vi "Sub_Initialize_LEMP.vi"(1 "Stiff":T2, 2 "Mass":T2) -> (0 "LEMP":T1)   [LabVIEW 2019]
uses:
  <vilib>/Analysis/Matrix/Datatypes/RealMatrix.ctl
  <vilib>/Analysis/Matrix/Numeric/Conversions/Matrix To Array - RM.vi
  <vilib>/Analysis/Matrix/Numeric/Conversions/Array To Matrix - RA2.vi
  <vilib>/Analysis/Matrix/NI_Matrix.lvlib
panel:
  # "Input"
  # "Output"
  # "This VI acquires the required input cluster for the Sub_online_LEMP_Update.vi, this VI calls on SciPy.linalg.eigh() due to issues with the standard \"General Eigenvalues and Eigenvectors.vi\" outputting inappropriately scaled eigenvectors for the LEMP. Additionally the Bitedness of this installation of LabVIEW does not match with Python so direct python calls were similarly unavailable. The workaround involved a saving the matrices in a text format command line calling the SciPy eigh function saving that output as a text file, then load the output file in to memory (See Sub_Python_cmd_eigh.vi, getEigenCommandPrompt.py , mass.lvm, stiff.lvm,eigenvalues.txt, eigenvectors.txt).\n\n              - Alexander Vereen AFRL Summer scholars 2022"
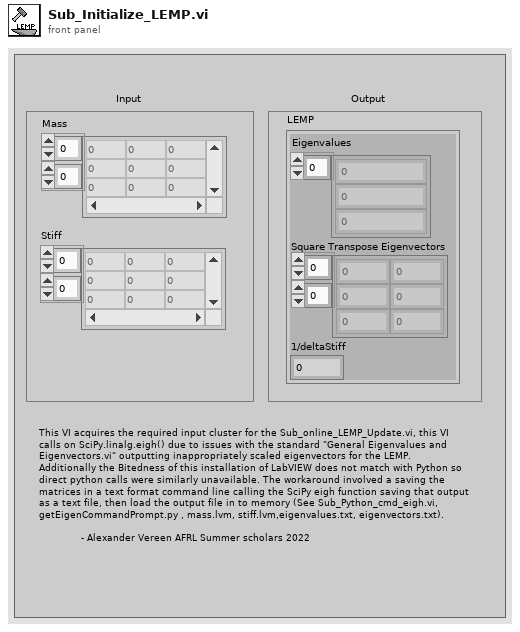
[diagram p1: front panel]
types:
  T1 = cluster{"Eigenvalues":dbl[], "Square Transpose Eigenvectors":dbl[][], "1/deltaStiff":dbl}
  T2 = typedef "NI_Matrix.lvlib/RealMatrix.ctl" = dbl[][]
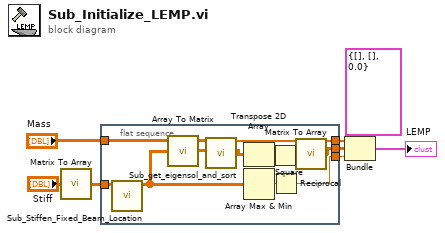
[diagram p0: block diagram]
diagram:
  n1 = call-poly <vilib>:"Matrix To Array.vi"("Real Matrix"="Stiff") -> ("Real 2D Array"=w7:dbl[][])
  n2 = flat-sequence {
    tunnel: [w18] -> w4
    tunnel: [w9] -> w3
    tunnel: [w14] -> w2
    tunnel: "Mass" -> [w13]
    tunnel: w7 -> [w11]
    frame #0 {
      n3 = call "Sub_Stiffen_Fixed_Beam_Location.vi"("Pre-BC Matrix"=w11) -> ("Post-BC Matrix"=w10:dbl[][])  [unwired: 10 in]
      n4 = call-poly <vilib>:"Array To Matrix.vi"("Real 2D Array"=w10) -> ("Real Matrix"=w12:T2)
      n5 = call "Sub_get_eigensol_and_sort.vi"("Mass"=w13, "Stiffness"=w12) -> ("Unsorted Eigenvalues"=w18:dbl[], "Unsorted Eigenvector Matrix"=w17:T2)  [unwired: 13 in, 3 out]
      n6 = Transpose 2D Array(2D array=w17) -> (transposed array=w19:T2)
      n7 = Array Max & Min(array=w10) -> (max value=w15:dbl)  [unwired: 3 out]
      n8 = Square(x=w19) -> (x^2=w16:T2)
      n9 = Reciprocal(x=w15) -> (1/x=w14:dbl)
      n10 = call-poly <vilib>:"Matrix To Array.vi"("Real Matrix"=w16) -> ("Real 2D Array"=w9:dbl[][])
    }
  }
  n11 = Bundle(cluster=T1 {"Eigenvalues"=[], "Square Transpose Eigenvectors"=[], "1/deltaStiff"=0.0} ("LEMP"), "Eigenvalues"=w4, "Square Transpose Eigenvectors"=w3, "1/deltaStiff"=w2) -> (→"LEMP":T1)
